vi "LT_unbundle_status.vi"(11 "Status word":T2) -> (2 "Remote has been activated":bool, 3 "Operation enabled":bool, 4 "enabled":T1(ring))   [LabVIEW 2019]
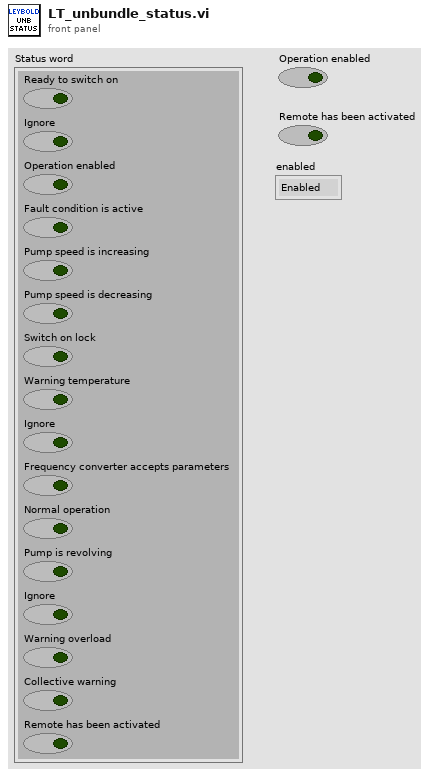
[diagram p1: front panel]
types:
  T1 = enum8{"Enabled", "Disabled", "Disabled and Grayed Out"}
  T2 = cluster{"Ready to switch on":bool, "Ignore":bool, "Operation enabled":bool, "Fault condition is active":bool, "Pump speed is increasing":bool, "Pump speed is decreasing":bool, "Switch on lock":bool, "Warning temperature":bool, "Ignore":bool, "Frequency converter accepts parameters":bool, "Normal operation":bool, "Pump is revolving":bool, "Ignore":bool, "Warning overload":bool, "Collective warning":bool, "Remote has been activated":bool}
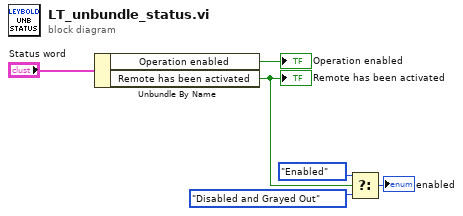
[diagram p0: block diagram]
diagram:
  n1 = Unbundle By Name("Status word") -> ("Operation enabled"=→"Operation enabled":bool, "Remote has been activated"=w2:bool)
  "Remote has been activated" <- w2
  n2 = Select(t=T1."Enabled" ("Disabled"), s=w2, f=T1."Disabled and Grayed Out" ("Disabled")) -> (s? t:f=→"enabled":T1)
